vi "Read Password file.vi"() -> (4 "Contents":string[][](array[string]))   [LabVIEW 2011]
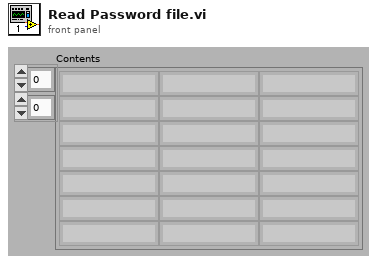
[diagram p1: front panel]
types:
  T1 = enum16{"open", "open or create", "create or replace", "create", "open (read only)"}
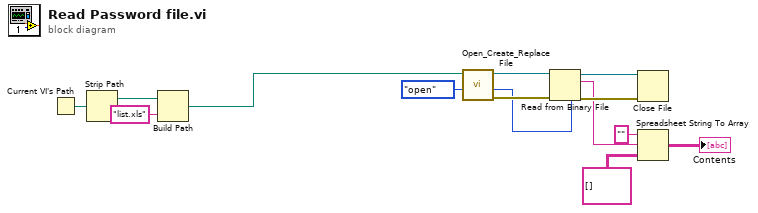
[diagram p0: block diagram]
diagram:
  n1 = Current VI's Path() -> (path=w4:path)
  n2 = Strip Path(path=w4) -> (stripped path=w3:path)  [unwired: 1 out]
  n3 = Build Path(base path=w3, name or relative path="list.xls") -> (appended path=w1:path)
  n4 = call <vilib>:"Open_Create_Replace File.vi"("function (open:0)"=T1."open", "file path"=w1) -> ("error out"=w14:errorcluster, "file size (bytes)"=w10:i32, "refnum"=w13:refnum<file>)  [unwired: 6 in, 1 out]
  n5 = Read from Binary File(8:w14, 10:w10, 11:w13) -> (0:w12:errorcluster, 2:w9:string, 3:w11:refnum<file>)  [unwired: 3 in, 1 out]
  n6 = Close File(refnum=w11, error in=w12) -> ()  [unwired: 2 out]
  n7 = Spreadsheet String To Array(format string="", spreadsheet string=w9, array type (2D Dbl)=string[][] []) -> (array=→"Contents":string[][])  [unwired: 1 in]
